vi "FTW-Test-JobScheduler.vi"() -> (0 "Test Result":errorcluster)   [LabVIEW 2015]
uses:
  src/actor/scheduler/FTW-Scheduler.lvclass
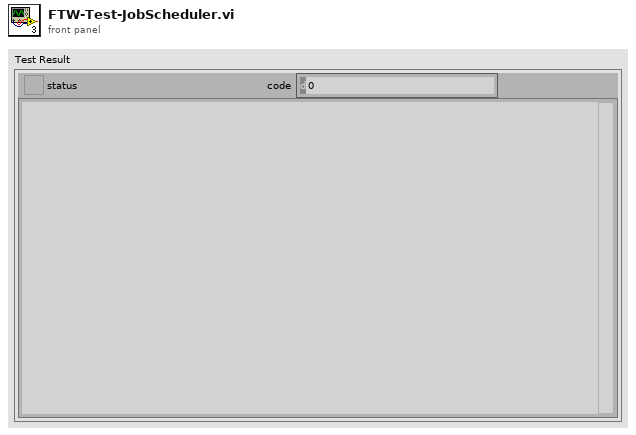
[diagram p1: front panel]
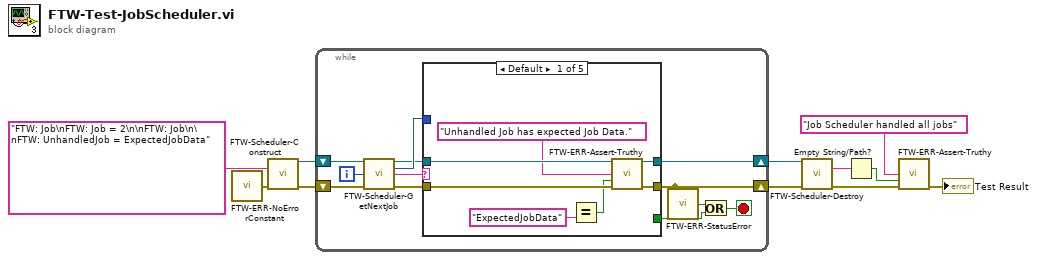
[diagram p0: block diagram]
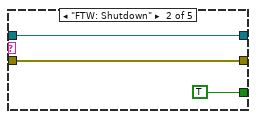
[diagram p2: hidden frame]
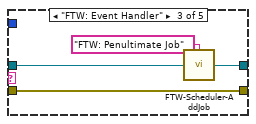
[diagram p3: hidden frame]
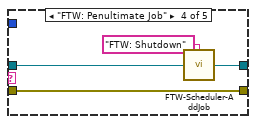
[diagram p4: hidden frame]
diagram:
  n1 = call "FTW-ERR-NoErrorConstant.vi"() -> ("no error"=w4:errorcluster)
  n2 = call "FTW-Scheduler-Construct.vi"("Initial Job Sequence"="FTW: Job\nFTW: Job = 2\n\nFTW: Job\n\nFTW: UnhandledJob = ExpectedJobData", "error in"=w4) -> ("FTW Job Scheduler"=w11:refnum<class "FTW-Scheduler.lvclass">, "error out"=w3:errorcluster)  [unwired: 12 in]
  n3 = while {
    shift-right: [w14] -> w9
    shift-left: w11 -> [w23]
    shift-right: [w17] -> w2
    shift-left: w3 -> [w22]
    i -> [w21]
    stop <- w15 stop-if-true
    n4 = call "FTW-Scheduler-GetNextJob.vi"("FTW Job Scheduler"=w23, "Jobs Performed"=w21, "error in"=w22) -> ("FTW Job Scheduler out"=w12:refnum<class "FTW-Scheduler.lvclass">, "Time til Next Scheduled Job"=w13:i32, "Current Job"=w20:string, "error out"=w18:errorcluster)  [unwired: 9 in]
    n5 = case shown="Default" w20 {
      tunnel: w12 -> [w29 w30 w35 w39 w41]
      tunnel: [_ TRUE _ _ _] -> w16
      tunnel: w18 -> [w27 w31 w36 w40 w42]
      tunnel: [w28 w31 w36 w40 w42] -> w17
      tunnel: [w29 w30 w34 w38 w41] -> w14
      tunnel: w13 -> [_ _ _ _ _]
      frame Default {
        n6 = Equal?(y="ExpectedJobData") -> (x = y?=w26:bool)  [unwired: 1 in]
        n7 = call "FTW-ERR-Assert-Truthy.vi"("Assertion"="Unhandled Job has expected Job Data.", "Assertion holds true?"=w26, "error in"=w27) -> ("error out"=w28:errorcluster)  [unwired: 12 in]
      }
      frame "FTW: Shutdown" {
      }
      frame "FTW: Event Handler" {
        n8 = call "FTW-Scheduler-AddJob.vi"("Add to Job Sequence"="FTW: Penultimate Job" ("Add Next in Sequence"), "FTW Job Scheduler"=w35) -> ("FTW Job Scheduler out"=w34:refnum<class "FTW-Scheduler.lvclass">)  [unwired: 2 in]
      }
      frame "FTW: Penultimate Job" {
        n9 = call "FTW-Scheduler-AddJob.vi"("Add to Job Sequence"="FTW: Shutdown" ("Add Next in Sequence"), "FTW Job Scheduler"=w39) -> ("FTW Job Scheduler out"=w38:refnum<class "FTW-Scheduler.lvclass">)  [unwired: 2 in]
      }
      frame "FTW: Job" {
      }
    }
    n10 = call "FTW-ERR-StatusError.vi"("error to check"=w17) -> ("Error?"=w19:bool)
    n11 = Or(x=w19, y=w16) -> (x .or. y?=w15:bool)
  }
  n12 = call "FTW-Scheduler-Destroy.vi"("FTW Job Scheduler"=w9, "error in"=w2) -> ("Remaining Jobs"=w8:string, "error out"=w1:errorcluster)  [unwired: 12 in]
  n13 = Empty String/Path?(string/path=w8) -> (empty?=w6:bool)
  n14 = call "FTW-ERR-Assert-Truthy.vi"("Assertion"="Job Scheduler handled all jobs", "Assertion holds true?"=w6, "error in"=w1) -> ("error out"=→"Test Result":errorcluster)  [unwired: 12 in]
